vi "ScreenLock.vi"   [LabVIEW 2018, in "OXYGEN.lvlib"]
uses:
  OXYGEN.lvlib
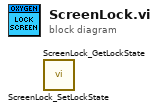
[diagram p0: block diagram]
diagram:
  n1 = call "ScreenLock_SetLockState.vi"() -> ()  [unwired: 9 in, 3 out]
  n2 = call "ScreenLock_GetLockState.vi"() -> ()  [unwired: 8 in, 4 out]
